vi "PRL SIGNAL Create Waveform by Interpolation.vi"(7 "Interpolate":bool, 10 "Data":dbl[](array[numeric]), 11 "Time Stamp":timestamp[](array[timestamp])) -> (3 "Waveform":waveform(dbl))   [LabVIEW 2013, in "PMU Recorder Light.lvlib"]
uses:
  PMU Recorder Light.lvlib
  <vilib>/Analysis/NI_AALBase.lvlib
  <vilib>/Analysis/1siggen.llb/Ramp Pattern by Samples.vi
  <vilib>/gmath/NI_Gmath.lvlib
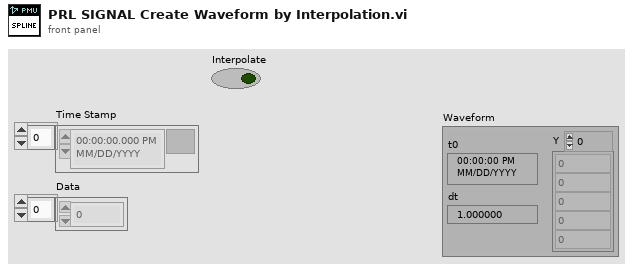
[diagram p1: front panel]
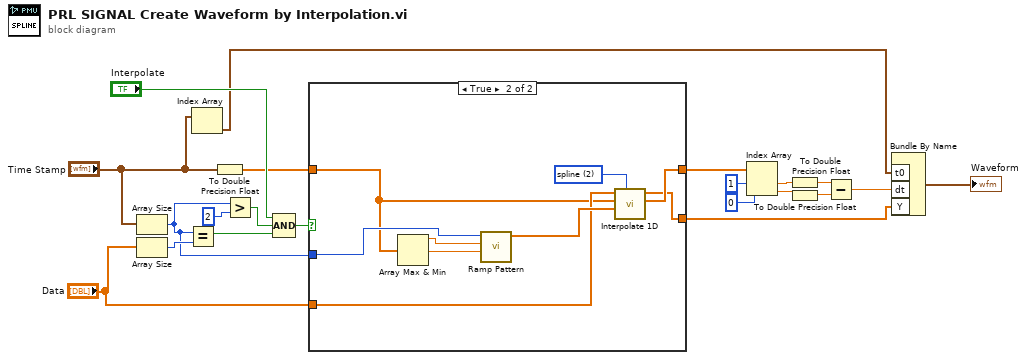
[diagram p0: block diagram]
diagram:
  n1 = Array Size(array="Time Stamp") -> (size(s)=w9:i32)
  n2 = Array Size(array="Data") -> (size(s)=w20:i32)
  n3 = Equal?(x=w9, y=w20) -> (x = y?=w17:bool)
  n4 = Index Array(array="Time Stamp") -> (element=w3:timestamp)  [unwired: 1 in]
  n5 = To Double Precision Float(number="Time Stamp") -> (double precision float=w6:dbl[])
  n6 = Greater?(x=w9, y=2) -> (0:w18:bool)
  n7 = Compound Arithmetic op=AND("Interpolate", w18, w17) -> (w7:bool)
  n8 = case shown="True" w7 {
    tunnel: w9 -> [_ w32]
    tunnel: w6 -> [w23 w26]
    tunnel: "Data" -> [w22 w28]
    tunnel: [w23 w25] -> w5
    tunnel: [w22 w24] -> w1
    frame False {
    }
    frame True {
      w27 = 2 items=["nearest", "linear", "spline", "cubic Hermite", "Lagrange"] ("method")
      n9 = Array Max & Min(array=w26) -> (max value=w31:dbl, min value=w30:dbl)  [unwired: 2 out]
      n10 = call-poly <vilib>:"Ramp Pattern.vi"("start"=w30, "end"=w31, "samples"=w32) -> ("Ramp Pattern"=w29:dbl[])  [unwired: 7 in, 1 out]
      n11 = call <vilib>:"Interpolate 1D.vi"("method"=w27, "xi"=w29, "X"=w26, "Y"=w28) -> ("xi used"=w25:dbl[], "yi"=w24:dbl[])  [unwired: 5 in, 1 out]
    }
  }
  n12 = Index Array(array=w5, index #1=1 ("index"), index #2=0 ("index")) -> (element #1=w12:dbl, element #2=w15:dbl)
  n13 = To Double Precision Float(number=w12) -> (double precision float=w13:dbl)
  n14 = To Double Precision Float(number=w15) -> (double precision float=w14:dbl)
  n15 = Subtract(x=w13, y=w14) -> (x-y=w2:dbl)
  n16 = Bundle By Name("t0"=w3, "dt"=w2, "Y"=w1) -> (→"Waveform":waveform(dbl))  [unwired: 1 in]
